vi "Channel_OpenWfms.vi"(8 "error in (no error)":errorcluster, 11 "Channel in":refnum<class "Channel.lvclass">) -> (0 "error out":errorcluster, 3 "Channel out":refnum<class "Channel.lvclass">)   [LabVIEW 2023, in "Channel.lvclass"]
doc: "Opens the waveform session during compilation from the System Explorer to the Engine in VeriStand"
uses:
  Channel.lvclass
  Channel.lvclass/Channel.ctl
  <vilib>/NI VeriStand/Custom Device API/Custom Device API.lvlib
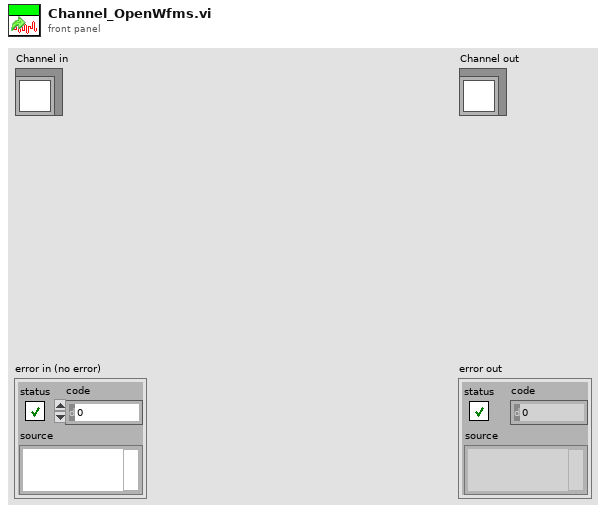
[diagram p1: front panel]
types:
  T1 = typedef "Custom Device API.lvlib/Data Reference.ctl" = i32
  T2 = typedef "Custom Device API.lvlib/Waveform Data Reference.ctl" = i32
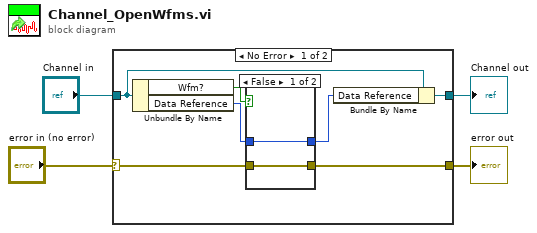
[diagram p0: block diagram]
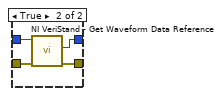
[diagram p2: hidden frame]
diagram:
  n1 = case shown="No Error" "error in (no error)" {
    selector: "error in (no error)" -> [w5 w19]
    tunnel: [w6 w19] -> w3
    tunnel: [w8 w18] -> w1
    tunnel: "Channel in" -> [w9 w18]
    frame No Error {
      n2 = Unbundle By Name(w9) -> ("Wfm?"=w11:bool, "Data Reference"=w10:T1)
      n3 = case shown="False" w11 {
        tunnel: w10 -> [w12 w17]
        tunnel: [w12 w16] -> w7
        tunnel: [w13 w15] -> w6
        tunnel: w5 -> [w13 w14]
        frame False {
        }
        frame True {
          n4 = call <vilib>:"NI VeriStand - Get Waveform Data Reference.vi"("error in (no error)"=w14, "Waveform Ref in"=w17) -> ("error out"=w15:errorcluster, "Waveform Data Reference"=w16:T2)  [unwired: 7 in, 1 out]
        }
      }
      n5 = Bundle By Name(cluster=w9, "Data Reference"=w7) -> (w8:refnum<class "Channel.lvclass">)
    }
    frame Error {
    }
  }
  "error out" <- w3
  "Channel out" <- w1
